vi "Main sandbox.vi"() -> ()   [LabVIEW 2018]
uses:
  RT/Type Defs/RT Status.ctl
  type defs/Comms loop variables.ctl
  Chris VIs/Incident logger/Incidents/Incident.lvclass
  Chris VIs/Incident logger/Incident logger.lvclass
  Chris VIs/Incident logger/Incidents/Quit/Quit.lvclass
panel:
  out "States":string[](array[string])
  out "data received":dbl[][](array[numeric])
  out "error stream":errorcluster
  out "RT Status":T1
  out "Relayed messages":string[](array[string])
  in  "Quit":bool
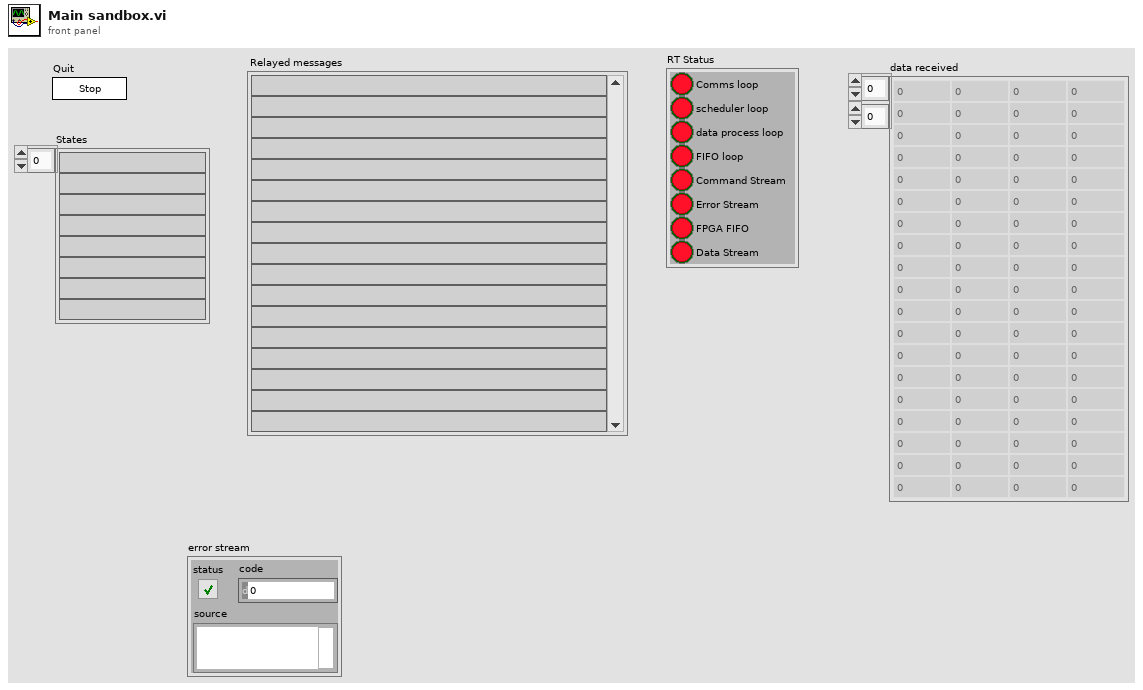
[diagram p1: front panel]
types:
  T1 = typedef "RT Status.ctl" = cluster{"Comms loop":bool, "scheduler loop":bool, "data process loop":bool, "FIFO loop":bool, "Command Stream":bool, "Error Stream":bool, "FPGA FIFO":bool, "Data Stream":bool}
  T2 = typedef "Comms loop variables.ctl" = cluster{"error stream":refnum<k21>, "Errors":refnum<class "Incident.lvclass">[], "command stream":refnum<k21>}
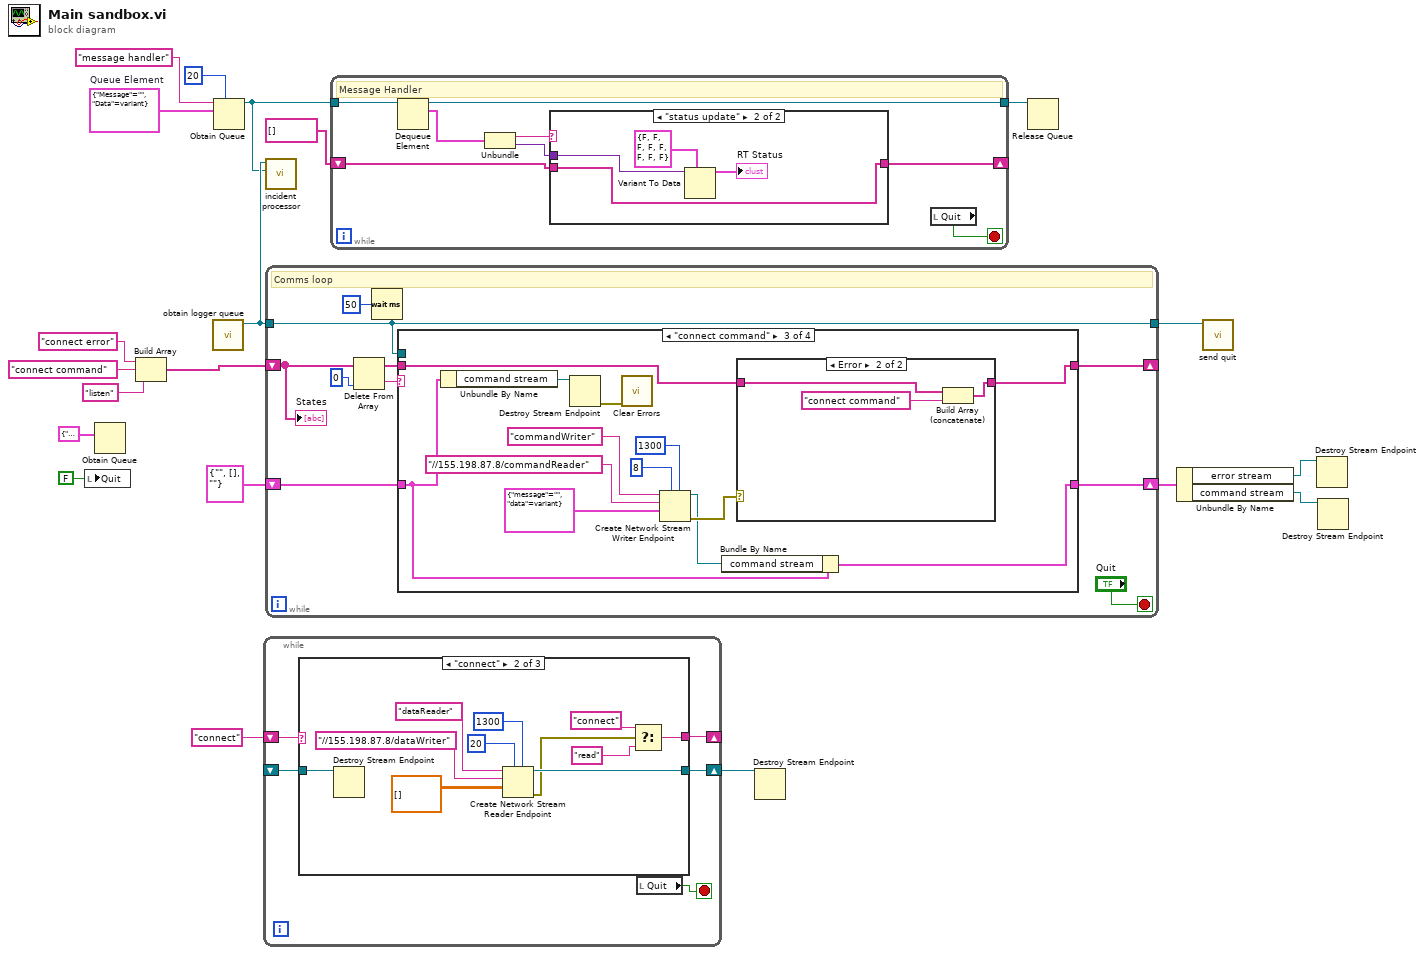
[diagram p0: block diagram]
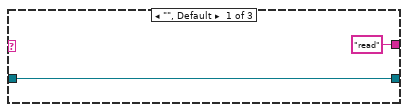
[diagram p2: hidden frame]
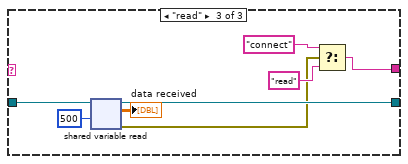
[diagram p3: hidden frame]
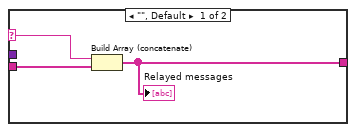
[diagram p4: hidden frame]
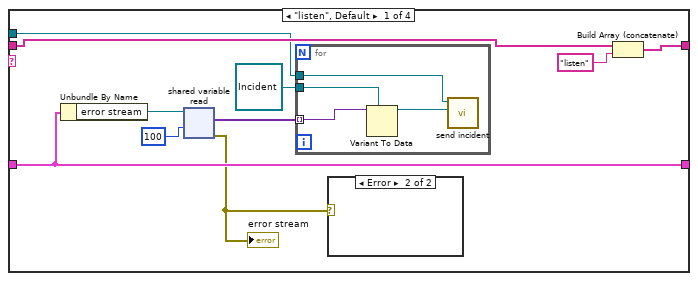
[diagram p5: hidden frame]
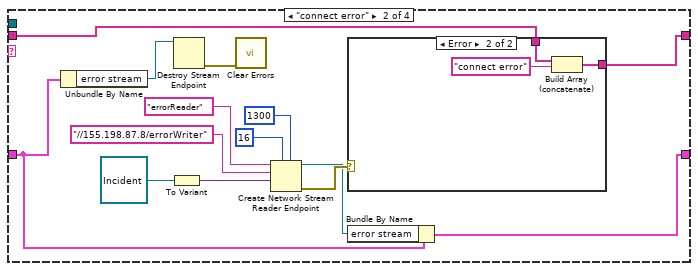
[diagram p7: hidden frame]
diagram:
  w13 = cluster{"Message":string, "Data":variant} {"Message"="", "Data"=variant}  # Queue Element
  n1 = local write "Quit"(FALSE ("Quit")) -> ()
  n2 = Obtain Queue(element data type=cluster{"message":string, "data":variant} {"message"="", "data"=variant}) -> ()  [unwired: 4 in, 3 out]
  n3 = Build Array("connect error", "connect command", "listen" ("element")) -> (w19:string[])
  n4 = call "obtain logger queue.vi"() -> ("Incident logger out"=w15:refnum<class "Incident logger.lvclass">)  [unwired: 10 in, 1 out]
  n5 = Obtain Queue(max queue size (-1, unlimited)=20, name (unnamed)="message handler", element data type=w13) -> (queue out=w11:refnum<queue>)  [unwired: 2 in, 2 out]
  n6 = while {
    shift-right: [w21] -> _
    shift-left: "connect" -> [w24]
    shift-right: [w23] -> w4
    shift-left: _ -> [w22]
    stop <- w25 stop-if-true
    n7 = case shown="\"connect\"" w24 {
      tunnel: [w27 w33 w44] -> w23
      tunnel: w22 -> [w27 w32 w46]
      tunnel: ["read" w28 w42] -> w21
      frame "", Default {
      }
      frame "connect" {
        n8 = Destroy Stream Endpoint(11:w32) -> ()  [unwired: 1 in, 1 out]
        n9 = Create Network Stream Reader Endpoint(5:1300 ("timeout in ms (-1)"), 7:20 ("reader buffer size"), 9:sgl[][] [], 10:"//155.198.87.8/dataWriter" ("writer url"), 11:"dataReader" ("reader name")) -> (0:w31:errorcluster, 3:w33:refnum<k21>)  [unwired: 2 in]
        n10 = Select(t="connect", s=w31, f="read") -> (s? t:f=w28:string)
      }
      frame "read" {
        n11 = shared-variable-read(w46, 500 ("timeout ms (-1)")) -> (w44:refnum<k21>, w40:errorcluster, →"data received":sgl[][])  [unwired: 1 in, 1 out]
        n12 = Select(t="connect", s=w40, f="read") -> (s? t:f=w42:string)
      }
    }
    n13 = local read "Quit"() -> (w25:bool)
  }
  n14 = call "incident processor.vi"("message queue"=w11, "Incident logger in"=w15) -> ()  [unwired: 10 in]
  n15 = while {
    shift-right: [w52] -> _
    shift-left: w19 -> [w56]
    shift-right: [w50] -> w3
    shift-left: T2 {"error stream"="", "Errors"=[], "command stream"=""} -> [w51]
    tunnel: w15 -> [w47]
    tunnel: [w47] -> w9
    stop <- "Quit" stop-if-true
    # "Comms loop"
    n16 = Delete From Array(array=w56, index=0) -> (deleted portion=w54:string, array with subset deleted=w53:string[])  [unwired: 1 in]
    n17 = Wait (ms)(milliseconds to wait=u32 50) -> ()  [unwired: 1 out]
    n18 = case shown="\"connect command\"" w54 {
      tunnel: w53 -> [w66 w72 w91 w106]
      tunnel: [w59 w71 w90 w106] -> w52
      tunnel: w51 -> [w63 w75 w94 w107]
      tunnel: [w63 w74 w93 w107] -> w50
      tunnel: w47 -> [w60 _ _ _]
      frame "listen", Default {
        n19 = Unbundle By Name(w63) -> ("error stream"=w65:refnum<k21>)
        n20 = shared-variable-read(w65, 100 ("timeout ms (-1)")) -> (w57:errorcluster, w61:variant[])  [unwired: 2 in, 2 out]
        "error stream" <- w57
        n21 = for {
          tunnel: refnum<class "Incident.lvclass"> refnum ("incident logger.lvlib:Incident.lvclass") -> [w70]
          tunnel: w61 -> [w69] mode=indexing
          tunnel: w60 -> [w67]
          n22 = Variant To Data(type=w70, Variant=w69) -> (data=w68:refnum<class "Incident.lvclass">)  [unwired: 1 in, 1 out]
          n23 = call "send incident.vi"("incident"=w68, "Incident logger in"=w67) -> ()  [unwired: 8 in, 2 out]
        }
        n24 = case shown="Error" w57 {
          frame No Error {
          }
          frame Error {
          }
        }
        n25 = Build Array (concatenate)(w66, "listen") -> (w59:string[])
      }
      frame "connect error" {
        n26 = Unbundle By Name(w75) -> ("error stream"=w77:refnum<k21>)
        n27 = To Variant(anything=refnum<class "Incident.lvclass"> refnum ("incident logger.lvlib:Incident.lvclass")) -> (Variant=w84:variant)
        n28 = Destroy Stream Endpoint(11:w77) -> (0:w76:errorcluster)  [unwired: 1 in]
        n29 = call <vilib>:"Clear Errors.vi"("error in (no error)"=w76) -> ()  [unwired: 5 in, 2 out]
        n30 = Create Network Stream Reader Endpoint(5:1300 ("timeout in ms (-1)"), 7:16 ("reader buffer size"), 9:w84, 10:"//155.198.87.8/errorWriter" ("writer url"), 11:"errorReader" ("reader name")) -> (0:w79:errorcluster, 3:w73:refnum<k21>)  [unwired: 2 in]
        n31 = case shown="Error" w79 {
          tunnel: w72 -> [w85 w88]
          tunnel: [w85 w87] -> w71
          frame No Error {
          }
          frame Error {
            n32 = Build Array (concatenate)(w88, "connect error" ("String")) -> (w87:string[])
          }
        }
        n33 = Bundle By Name(cluster=w75, "error stream"=w73) -> (w74:T2)
      }
      frame "connect command" {
        n34 = Unbundle By Name(w94) -> ("command stream"=w96:refnum<k21>)
        n35 = Destroy Stream Endpoint(11:w96) -> (0:w95:errorcluster)  [unwired: 1 in]
        n36 = call <vilib>:"Clear Errors.vi"("error in (no error)"=w95) -> ()  [unwired: 5 in, 2 out]
        n37 = Create Network Stream Writer Endpoint(5:1300 ("timeout in ms (-1)"), 7:8 ("reader buffer size"), 9:cluster{"message":string, "data":variant} {"message"="", "data"=variant}, 10:"//155.198.87.8/commandReader" ("writer url"), 11:"commandWriter" ("reader name")) -> (0:w98:errorcluster, 3:w92:refnum<k21>)  [unwired: 2 in]
        n38 = Bundle By Name(cluster=w94, "command stream"=w92) -> (w93:T2)
        n39 = case shown="Error" w98 {
          tunnel: w91 -> [w102 w105]
          tunnel: [w102 w103] -> w90
          frame No Error {
          }
          frame Error {
            n40 = Build Array (concatenate)(w105, "connect command" ("String")) -> (w103:string[])
          }
        }
      }
      frame "send command" {
      }
    }
    "States" <- w56
  }
  n41 = while {
    tunnel: w11 -> [w115]
    shift-right: [w111] -> _
    shift-left: string[] [] -> [w112]
    tunnel: [w109] -> w8
    stop <- w110 stop-if-true
    # "Message Handler"
    n42 = Dequeue Element(queue=w115) -> (queue out=w109:refnum<queue>, element=w114:cluster{"Message":string, "Data":variant})  [unwired: 2 in, 2 out]
    n43 = Unbundle(w114) -> ("Message"=w113:string, "Data"=w108:variant)
    n44 = case shown="\"status update\"" w113 {
      selector: w113 -> [w117 _]
      tunnel: w112 -> [w118 w122]
      tunnel: [w116 w122] -> w111
      tunnel: w108 -> [_ w121]
      frame "", Default {
        n45 = Build Array (concatenate)(w117, w118) -> (w116:string[])
        "Relayed messages" <- w116
      }
      frame "status update" {
        n46 = Variant To Data(type=T1 {"Comms loop"=FALSE, "scheduler loop"=FALSE, "data process loop"=FALSE, "FIFO loop"=FALSE, "Command Stream"=FALSE, "Error Stream"=FALSE, "FPGA FIFO"=FALSE, "Data Stream"=FALSE} ("RT Status"), Variant=w121) -> (data=→"RT Status":T1)  [unwired: 1 in, 1 out]
      }
    }
    n47 = local read "Quit"() -> (w110:bool)
  }
  n48 = Destroy Stream Endpoint(11:w4) -> ()  [unwired: 1 in, 1 out]
  n49 = Release Queue(queue=w8) -> ()  [unwired: 2 in, 3 out]
  n50 = Unbundle By Name(w3) -> ("error stream"=w2:refnum<k21>, "command stream"=w1:refnum<k21>)
  n51 = call "send quit.vi"("incident logger"=w9) -> ()  [unwired: 10 in, 1 out]
  n52 = Destroy Stream Endpoint(11:w2) -> ()  [unwired: 1 in, 1 out]
  n53 = Destroy Stream Endpoint(11:w1) -> ()  [unwired: 1 in, 1 out]
